vi "CloseBGImages.vi"(8 "error in (no error)":errorcluster, 11 "BGImages":T1) -> (0 "error out":errorcluster)   [LabVIEW 2013, in "MagAnalysis_Online.lvclass"]
uses:
  MagAnalysis_Online.lvclass
  bgImages_tyudef.ctl
  IMAQ Image.ctl
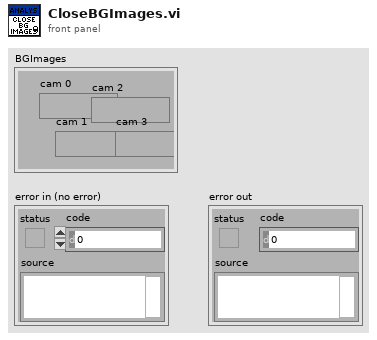
[diagram p1: front panel]
types:
  T1 = typedef "bgImages_tyudef.ctl" = cluster{"cam 0":T2, "cam 1":T2, "cam 2":T2, "cam 3":T2}
  T2 = typedef "IMAQ Image.ctl" = refnum<image>
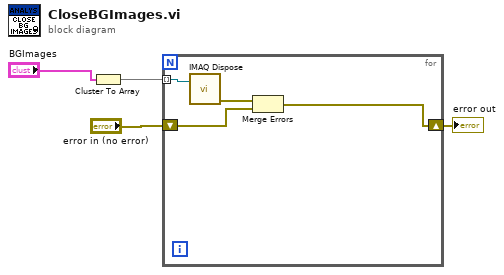
[diagram p0: block diagram]
diagram:
  n1 = Cluster To Array(cluster="BGImages") -> (array=w2:T2[])
  n2 = for {
    tunnel: w2 -> [w8] mode=indexing
    shift-right: [w5] -> w4
    shift-left: "error in (no error)" -> [w6]
    n3 = call "IMAQ Dispose"("Image"=w8) -> ("error out"=w7:errorcluster)  [unwired: 5 in]
    n4 = Merge Errors(w7, w6) -> (w5:errorcluster)
  }
  "error out" <- w4
